vi "Parse Measurement(fixed).vi"(6 "Measurement Line":string) -> (13 "Voltage":dbl, 14 "Measure String Array":string[](array[string]), 15 "Frequency":dbl, 16 "Capacitance":dbl format="%#_10f", 17 "Loss":dbl format="%#_10f", 18 "Units":i32(ring) items=["", "nanosiemens", "dissipation factor", "kilohms", "gigohms", "loss vector (jpF)"], 19 "Loss Greater Than":bool)   [LabVIEW 2017, in "Andeen-Hagerling 2700.lvlib"]
doc: "This VI parses a text line of measurement results from the bridge. Measurement results are dependent on the labelling parameter of Format and the Field parameters. Boolean inputs are provided to represent these parameters. These only need to be set if the the Format or Field are not set as in the Default Instrument Setup VI."
uses:
  <instrlib>/Andeen-Hagerling 2700/Andeen-Hagerling 2700.lvlib
panel:
  # "Measurement Results"
  # "Format Parameter"
  # "Field Parameters"
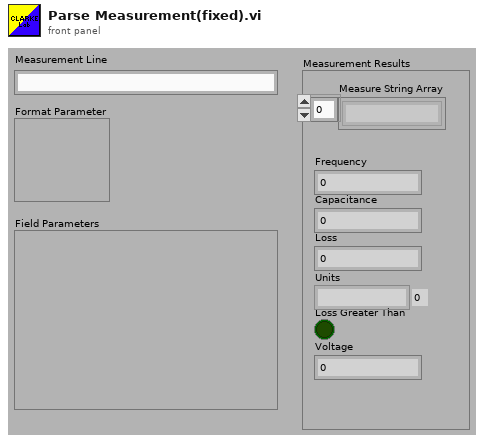
[diagram p1: front panel]
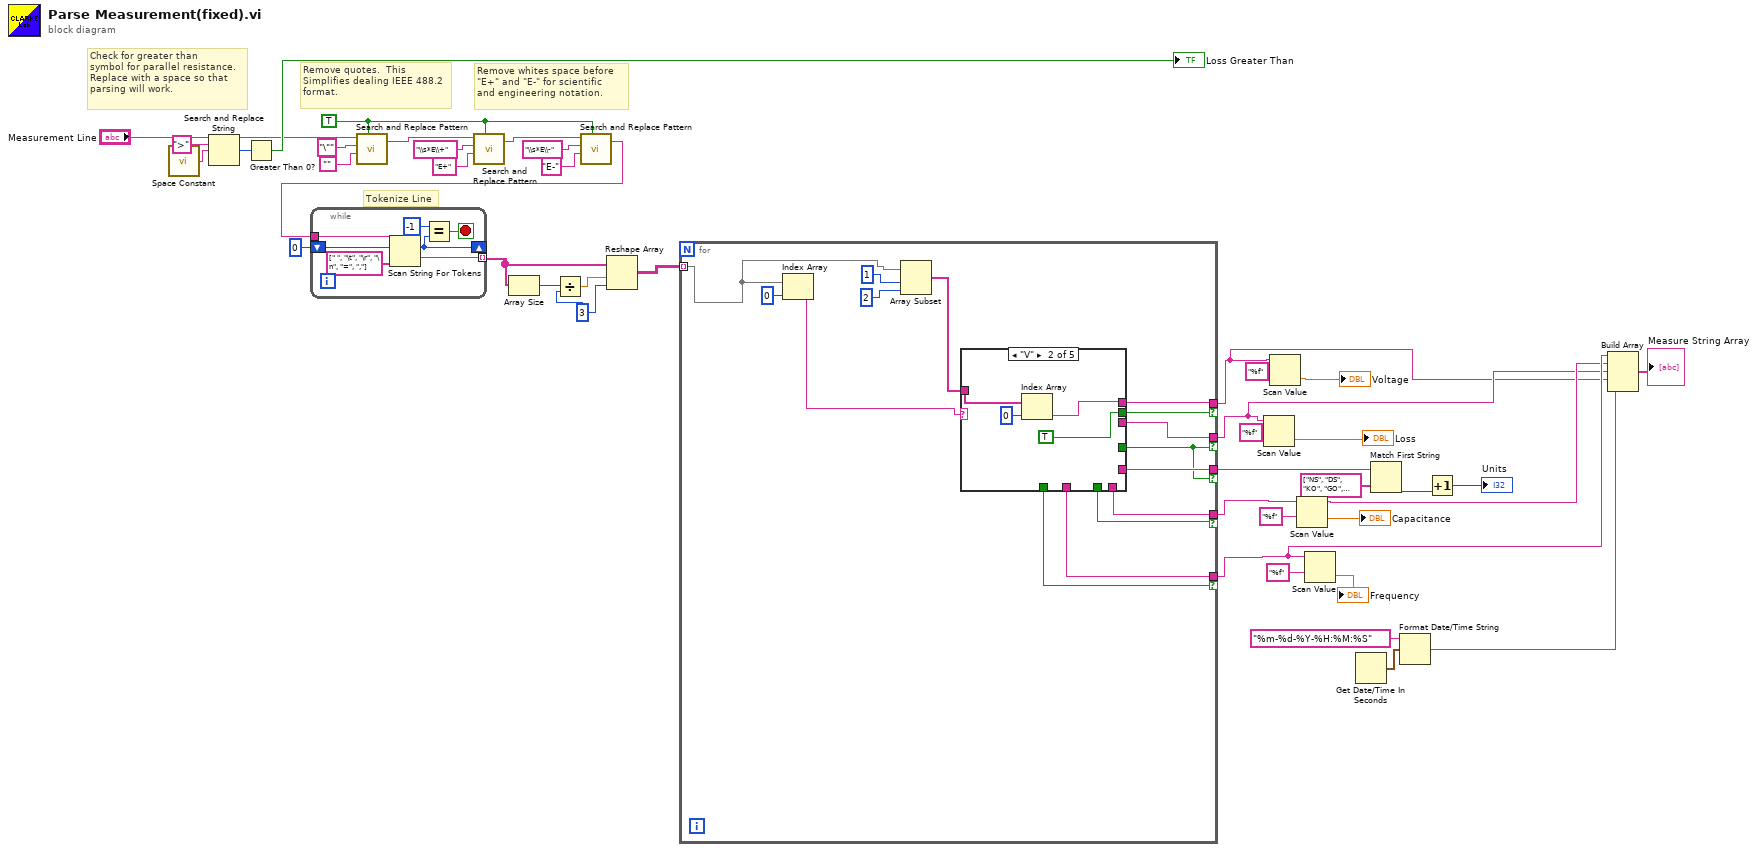
[diagram p0: block diagram]
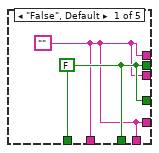
[diagram p2: hidden frame]
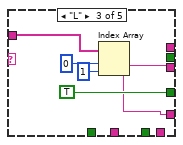
[diagram p3: hidden frame]
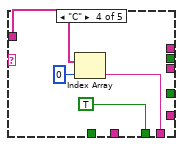
[diagram p4: hidden frame]
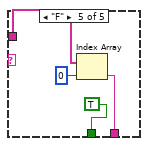
[diagram p5: hidden frame]
diagram:
  w22 = 3 ("dimension size")
  w28 = TRUE ("replace all? (F)")
  # "Remove quotes.  This\nSimplifies dealing IEEE 488.2\nformat."
  # "Remove whites space before\n\"E+\" and \"E-\" for scientific\nand engineering notation."
  # "Tokenize Line"
  # "Check for greater than\nsymbol for parallel resistance.\nReplace with a space so that\nparsing will work."
  n1 = call <vilib>:"Space Constant.vi"() -> ("String"=w40:string)
  n2 = Search and Replace String(input string="Measurement Line", search string=">", replace string=w40) -> (result string=w27:string, number of replacements=w41:i32)  [unwired: 5 in, 2 out]
  n3 = Greater Than 0?(x=w41) -> (x > 0?=→"Loss Greater Than":bool)
  n4 = call <vilib>:"Search and Replace Pattern.vi"("string"=w27, "regular expression (\"\")"="\"" ("regular expression (\"\")"), "replace string (\"\")"="", "replace all? (F)"=w28) -> ("result string"=w31:string)  [unwired: 1 in, 1 out]
  n5 = call <vilib>:"Search and Replace Pattern.vi"("string"=w31, "regular expression (\"\")"="\\s*E\\+" ("regular expression (\"\")"), "replace string (\"\")"="E+" ("replace string (\"\")"), "replace all? (F)"=w28) -> ("result string"=w32:string)  [unwired: 1 in, 1 out]
  n6 = call <vilib>:"Search and Replace Pattern.vi"("string"=w32, "regular expression (\"\")"="\\s*E\\-" ("regular expression (\"\")"), "replace string (\"\")"="E-" ("replace string (\"\")"), "replace all? (F)"=w28) -> ("result string"=w26:string)  [unwired: 1 in, 1 out]
  n7 = while {
    tunnel: [w48] -> w24 mode=indexing
    tunnel: w26 -> [w47]
    shift-right: [w45] -> _
    shift-left: 0 ("token index") -> [w46]
    stop <- w49 stop-if-true
    n8 = Scan String For Tokens(6:string[] [" ", "\t", "\r", "\n", "=", ","] ("delimiters (\\s,\\t,\\r,\\n)"), 8:w46, 9:w47) -> (1:w48:string, 2:w45:i32)  [unwired: 3 in, 2 out]
    n9 = Equal?(x=-1 ("y"), y=w45) -> (x = y?=w49:bool)
  }
  n10 = Array Size(array=w24) -> (size(s)=w25:i32)
  n11 = Divide(x=w25, y=w22) -> (x/y=w23:dbl)
  n12 = Reshape Array(w24, w23, w22) -> (w21:string[][])
  n13 = for {
    tunnel: w21 -> [w63] mode=indexing
    tunnel: [w58] -> w4 if=w53
    tunnel: [w57] -> w5 if=w50
    tunnel: [w56] -> w6 if=w51
    tunnel: [w55] -> w7 if=w52
    tunnel: [w54] -> w9 if=w50
    n14 = Index Array(array=w63, index=0) -> (element=w60:string)
    n15 = Array Subset(array=w63, index=1, length=2 ("index")) -> (w59:string[])
    n16 = case shown="\"V\"" w60 {
      tunnel: w59 -> [_ w69 w75 w78 w82]
      tunnel: [w65 w68 _ _ _] -> w58
      tunnel: [w65 _ w74 _ _] -> w57
      tunnel: [w65 _ _ w79 _] -> w56
      tunnel: [w65 _ _ _ w83] -> w55
      tunnel: [w65 _ w71 _ _] -> w54
      tunnel: [w66 TRUE _ _ _] -> w53
      tunnel: [w66 _ TRUE _ _] -> w50
      tunnel: [w66 _ _ TRUE _] -> w51
      tunnel: [w66 _ _ _ TRUE] -> w52
      frame "False", Default {
        w65 = ""
        w66 = FALSE
      }
      frame "V" {
        n17 = Index Array(array=w69, index=0) -> (element=w68:string)
      }
      frame "L" {
        n18 = Index Array(array=w75, index #1=0 ("index"), index #2=1 ("index")) -> (element #1=w74:string, element #2=w71:string)
      }
      frame "C" {
        n19 = Index Array(array=w78, index=0) -> (element=w79:string)
      }
      frame "F" {
        n20 = Index Array(array=w82, index=0) -> (element=w83:string)
      }
    }
  }
  n21 = Scan Value(string=w5, format string="%f") -> (value=→"Loss":dbl)  [unwired: 1 in, 1 out]
  n22 = Scan Value(string=w4, format string="%f") -> (value=→"Voltage":dbl)  [unwired: 1 in, 1 out]
  n23 = Scan Value(string=w6, format string="%f") -> (value=→"Capacitance":dbl)  [unwired: 1 in, 1 out]
  n24 = Scan Value(string=w7, format string="%f") -> (value=→"Frequency":dbl)  [unwired: 1 in, 1 out]
  n25 = Get Date/Time In Seconds() -> (seconds since 1Jan1904=w3:timestamp)
  n26 = Match First String(2:string[] ["NS", "DS", "KO", "GO", "JP"] ("string array"), 3:w9) -> (0:w19:i32)  [unwired: 1 out]
  n27 = Format Date/Time String(time format string (%c)="%m-%d-%Y-%H:%M:%S", seconds (now)=w3) -> (date/time string=w1:string)  [unwired: 1 in]
  n28 = Increment(x=w19) -> (x+1=→"Units":i32)
  n29 = Build Array(w7, w6, w5, w4, w1) -> (→"Measure String Array":string[])
